vi "Open and Deploy RT Sequence blocking call.vi"(4 "Target (\"\": Auto-assign)":string, 5 "Timeout (ms)":dbl=10000.0, 6 "Gateway IP Address":string, 7 "Sequence File Path":path, 8 "ParamTypes":string[](array[string]), 9 "ParamValues":string[](array[string]), 10 "ParamNames":string[](array[string]), 11 "Sequence Context":refnum<k7>) -> (0 "error out":errorcluster, 2 "Report Text":string)   [LabVIEW 2015, in "RTSequenceVIs.lvlib"]
uses:
  RTSequenceVIs.lvlib
  <vilib>/NI Veristand/Execution/SequenceExecutionInterface/Sequence Execution State.ctl
  NationalInstruments.VeriStand.DataTypes
  <vilib>/NI Veristand/Execution/SequenceExecutionInterface/NI_VS Sequence Execution Interface.lvlib
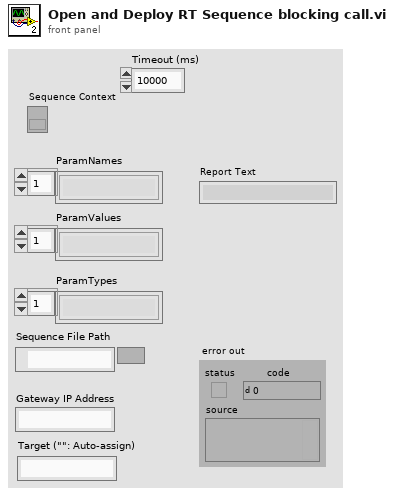
[diagram p1: front panel]
types:
  T1 = typedef "NI_VS Sequence Execution Interface.lvlib/Sequence Input Assignment Ref.ctl" = refnum<k24>
  T2 = typedef "NI_VS Sequence Execution Interface.lvlib/Sequence Call Ref.ctl" = refnum<k24>
  T3 = typedef "NI_VS Sequence Execution Interface.lvlib/Stimulus Profile Session Ref.ctl" = refnum<k24>
  T4 = typedef "TestStand - Status Monitor.ctl" = cluster{"Sequence Context":refnum<k7>, "Execution":refnum<k7>, "Termination Monitor":refnum<k7>}
  T5 = typedef "NI_VS Sequence Execution Interface.lvlib/Sequence Execution State.ctl" = enum16{"Idle", "Running", "SingleStepping", "Paused", "Stopped"}
  T6 = typedef "NI_VS Sequence Execution Interface.lvlib/Data Value Ref.ctl" = refnum<k24>
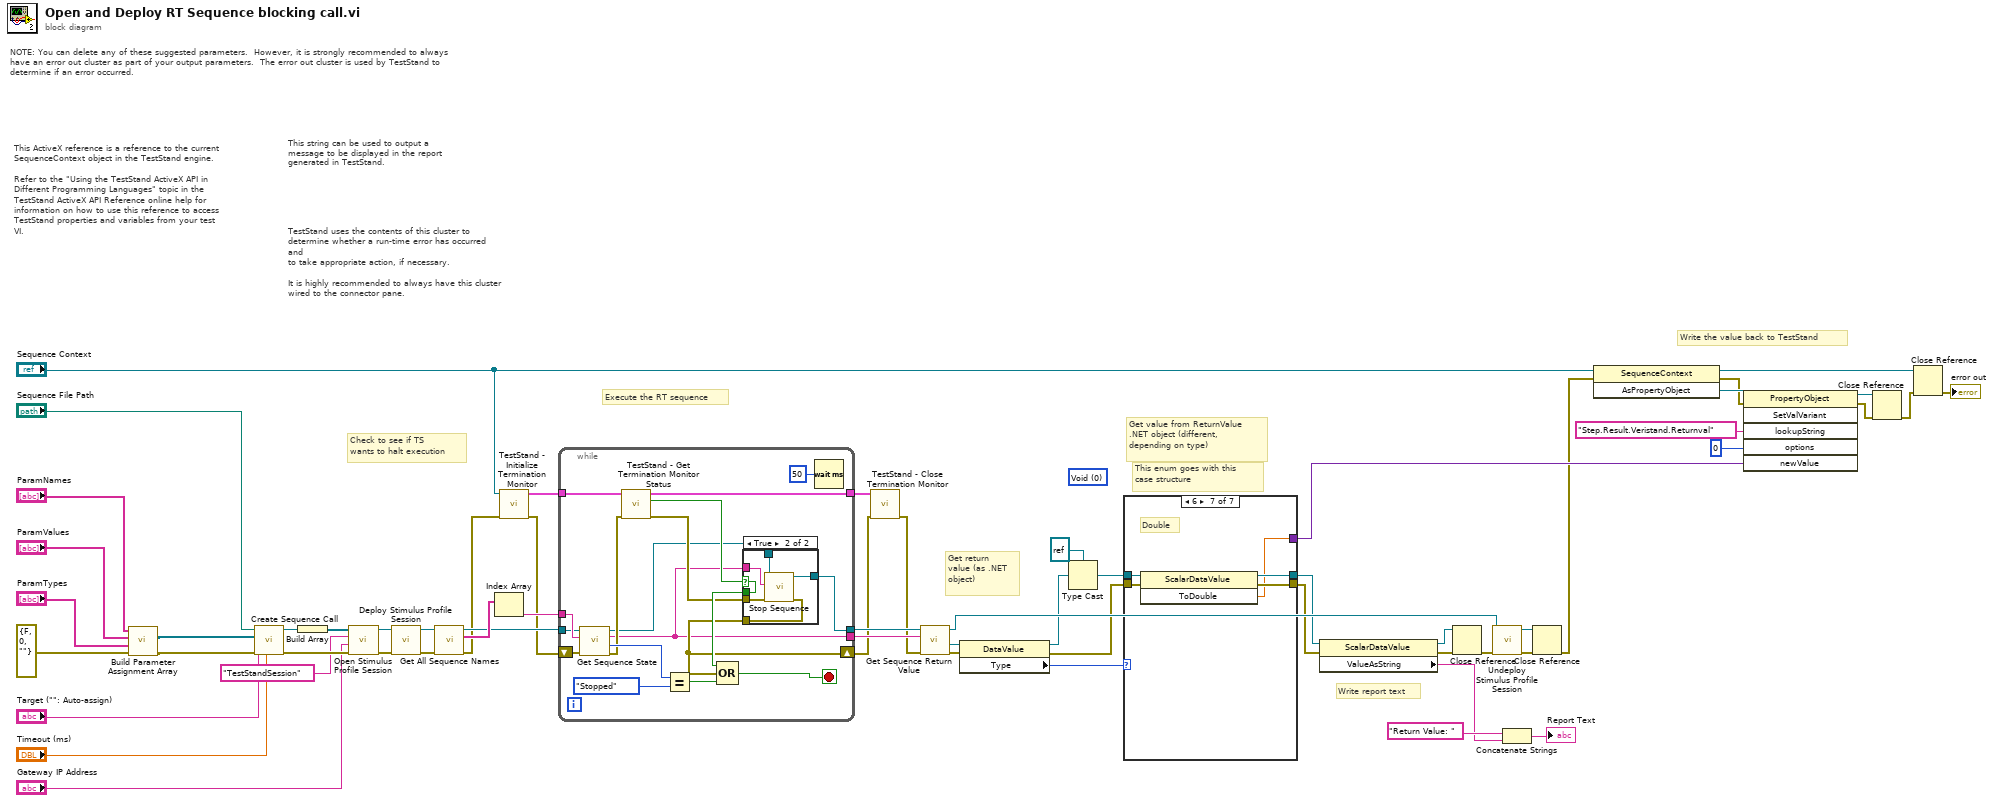
[diagram p0: block diagram]
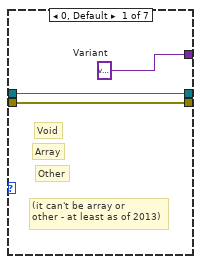
[diagram p2: hidden frame]
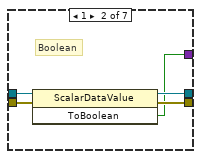
[diagram p3: hidden frame]
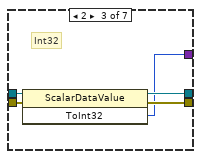
[diagram p4: hidden frame]
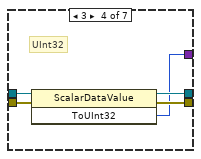
[diagram p5: hidden frame]
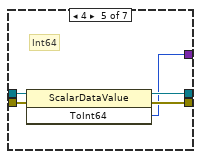
[diagram p6: hidden frame]
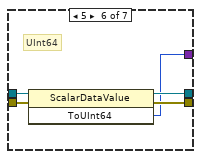
[diagram p7: hidden frame]
diagram:
  (unwired) 0 items=["Void", "Boolean", "Int32", "UInt32", "Int64", "UInt64", "Double", "Array"] ("Type")
  # "Check to see if TS\nwants to halt execution"
  # "Get value from ReturnValue\n.NET object (different, \ndepending on type)"
  # "Get return \nvalue (as .NET\nobject)"
  # "Write report text"
  # "Write the value back to TestStand"
  # "This enum goes with this \ncase structure"
  # "Execute the RT sequence"
  # "TestStand uses the contents of this cluster to\ndetermine whether a run-time error has occurred and\nto take appropriate action, if necessary.\n\nIt is highly recommended to always have this cluster\nwired to the connector pane."
  # "This string can be used to output a\nmessage to be displayed in the report\ngenerated in TestStand."
  # "NOTE: You can delete any of these suggested parameters.  However, it is strongly recommended to always have an error out cluster as part of your output parameters.  The error out cluster is used by TestStand to determine if an error occurred."
  # "This ActiveX reference is a reference to the current\nSequenceContext object in the TestStand engine.\n\nRefer to the \"Using the TestStand ActiveX API in\nDifferent Programming Languages\" topic in the \nTestStand ActiveX API Reference online help for\ninformation on how to use this reference to access\nTestStand properties and variables from your test VI."
  n1 = call "Build Parameter Assignment Array.vi"("error in (no error)"=errorcluster {"status"=FALSE, "code"=0, "source"=""}, "ParamTypes"="ParamTypes", "ParamValues"="ParamValues", "ParamNames"="ParamNames") -> ("error out"=w6:errorcluster, "Sequence Parameter Assignment refs"=w1:T1[])  [unwired: 6 in]
  n2 = call <vilib>:"Create Sequence Call.vi"("Timeout ms (10000)"="Timeout (ms)", "error in (no error)"=w6, "Target (\"\": Auto-assign)"="Target (\"\": Auto-assign)", "Parameter Assignments"=w1, "Sequence File Path"="Sequence File Path") -> ("error out"=w59:errorcluster, "Sequence Call Ref"=w53:T2)  [unwired: 5 in]
  n3 = Build Array(w53) -> (w57:T2[])
  n4 = call <vilib>:"Open Stimulus Profile Session.vi"("error in (no error)"=w59, "Gateway IP Address (\"\": localhost)"="Gateway IP Address", "Session Name"="TestStandSession", "Sequence Calls"=w57) -> ("error out"=w55:errorcluster, "Session Ref"=w56:T3)  [unwired: 6 in]
  n5 = call <vilib>:"Deploy Stimulus Profile Session.vi"("error in (no error)"=w55, "Session Ref in"=w56) -> ("error out"=w52:errorcluster, "Session Ref out"=w51:T3)  [unwired: 7 in, 1 out]
  n6 = call <vilib>:"Get All Sequence Names.vi"("error in (no error)"=w52, "Session Ref in"=w51) -> ("error out"=w15:errorcluster, "Sequence Names out"=w50:string[], "Session Ref out"=w48:T3)  [unwired: 7 in]
  n7 = Index Array(array=w50) -> (element=w49:string)  [unwired: 1 in]
  n8 = call <vilib>:"TestStand - Initialize Termination Monitor.vi"("error in (no error)"=w15, "Sequence Context In"="Sequence Context") -> ("error out"=w14:errorcluster, "Status Monitor Out"=w13:T4)  [unwired: 8 in]
  n9 = while {
    tunnel: w49 -> [w77]
    tunnel: w48 -> [w76]
    shift-right: [w63] -> w11
    shift-left: w14 -> [w75]
    tunnel: [w60] -> w44
    tunnel: [w62] -> w47
    tunnel: w13 -> [w69]
    tunnel: [w67] -> w12
    stop <- w71 stop-if-true
    n10 = call <vilib>:"Get Sequence State.vi"("error in (no error)"=w75, "Sequence Name"=w77, "Session Ref in"=w76) -> ("error out"=w68:errorcluster, "State"=w74:T5, "Sequence Name out"=w62:string, "Session Ref out"=w61:T3)  [unwired: 5 in]
    n11 = call <vilib>:"TestStand - Get Termination Monitor Status.vi"("error in (no error)"=w68, "Status Monitor In"=w69) -> ("error out"=w64:errorcluster, "Terminating or Aborting"=w66:bool, "Status Monitor Out"=w67:T4)  [unwired: 7 in]
    n12 = Equal?(x=w74, y=Sequence_Execution_State."Stopped" ("State")) -> (x = y?=w72:bool)
    n13 = case shown="True" w66 {
      selector: w66 -> [w80 w86]
      tunnel: [w80 w86] -> w65
      tunnel: w64 -> [w79 w85]
      tunnel: [w79 w84] -> w63
      tunnel: w62 -> [_ w83]
      tunnel: w61 -> [w78 w82]
      tunnel: [w78 w81] -> w60
      frame False {
      }
      frame True {
        n14 = call <vilib>:"Stop Sequence.vi"("error in (no error)"=w85, "Sequence Name"=w83, "Session Ref in"=w82) -> ("error out"=w84:errorcluster, "Session Ref out"=w81:T3)  [unwired: 6 in, 1 out]
      }
    }
    n15 = Compound Arithmetic op=OR(w65, w63, w72) -> (w71:bool)
    n16 = Wait (ms)(milliseconds to wait=u32 50 ("millisecond multiple")) -> ()  [unwired: 1 out]
  }
  n17 = call <vilib>:"TestStand - Close Termination Monitor.vi"("error in (no error)"=w11, "Status Monitor In"=w12) -> ("error out"=w10:errorcluster)  [unwired: 9 in]
  n18 = call <vilib>:"Get Sequence Return Value.vi"("error in (no error)"=w10, "Sequence Name"=w47, "Session Ref in"=w44) -> ("error out"=w38:errorcluster, "Data Value Ref"=w28:T6, "Session Ref out"=w43:T3)  [unwired: 5 in, 1 out]
  n19 = property class="DataValue"(reference=w28, error in=w38) -> (reference out=w36:T6, error out=w37:errorcluster, "Type"=w39:i32)
  n20 = Type Cast(type=refnum<k24> refnum ("Node"), x=w36) -> (*(type *) &x=w45:refnum<k24>)
  n21 = case shown="6" w39 {
    tunnel: w45 -> [w89 w94 w99 w104 w109 w114 w119]
    tunnel: [w88 w93 w97 w101 w106 w111 w116] -> w26
    tunnel: [w89 w92 w96 w102 w107 w112 w117] -> w27
    tunnel: w37 -> [w88 w91 w98 w103 w108 w113 w118]
    tunnel: [w87 w90 w95 w100 w105 w110 w115] -> w35
    frame 0, Default {
      w87 = variant  # Variant
      # "(it can't be array or \nother - at least as of 2013)"
      # "Other"
      # "Array"
      # "Void"
    }
    frame 1 {
      # "Boolean"
      n22 = invoke class="ScalarDataValue" method="ToBoolean"(reference=w94, error in=w91) -> (reference out=w92:refnum<k24>, error out=w93:errorcluster, "ToBoolean"=w90:bool)  [unwired: 1 in]
    }
    frame 2 {
      # "Int32"
      n23 = invoke class="ScalarDataValue" method="ToInt32"(reference=w99, error in=w98) -> (reference out=w96:refnum<k24>, error out=w97:errorcluster, "ToInt32"=w95:i32)  [unwired: 1 in]
    }
    frame 3 {
      # "UInt32"
      n24 = invoke class="ScalarDataValue" method="ToUInt32"(reference=w104, error in=w103) -> (reference out=w102:refnum<k24>, error out=w101:errorcluster, "ToUInt32"=w100:u32)  [unwired: 1 in]
    }
    frame 4 {
      # "Int64"
      n25 = invoke class="ScalarDataValue" method="ToInt64"(reference=w109, error in=w108) -> (reference out=w107:refnum<k24>, error out=w106:errorcluster, "ToInt64"=w105:i64)  [unwired: 1 in]
    }
    frame 5 {
      # "UInt64"
      n26 = invoke class="ScalarDataValue" method="ToUInt64"(reference=w114, error in=w113) -> (reference out=w112:refnum<k24>, error out=w111:errorcluster, "ToUInt64"=w110:u64)  [unwired: 1 in]
    }
    frame 6 {
      # "Double"
      n27 = invoke class="ScalarDataValue" method="ToDouble"(reference=w119, error in=w118) -> (reference out=w117:refnum<k24>, error out=w116:errorcluster, "ToDouble"=w115:dbl)  [unwired: 1 in]
    }
  }
  n28 = property class="ScalarDataValue"(reference=w27, error in=w26) -> (reference out=w25:refnum<k24>, error out=w24:errorcluster, "ValueAsString"=w17:string)
  n29 = Close Reference(reference=w25, error in (no error)=w24) -> (error out=w42:errorcluster)
  n30 = call <vilib>:"Undeploy Stimulus Profile Session.vi"("error in (no error)"=w42, "Session Ref in"=w43) -> ("error out"=w23:errorcluster, "Session Ref out"=w22:T3)  [unwired: 8 in]
  n31 = Concatenate Strings("Return Value: ", w17) -> (→"Report Text":string)
  n32 = Close Reference(reference=w22, error in (no error)=w23) -> (error out=w21:errorcluster)
  n33 = invoke class="SequenceContext" method="AsPropertyObject"(reference="Sequence Context", error in=w21) -> (reference out=w32:refnum<k7>, error out=w30:errorcluster, "AsPropertyObject"=w41:refnum<k7>)  [unwired: 1 in]
  n34 = invoke class="PropertyObject" method="SetValVariant"(reference=w41, error in=w30, "lookupString"="Step.Result.Veristand.Returnval", "options"=0, "newValue"=w35) -> (reference out=w34:refnum<k7>, error out=w33:errorcluster)  [unwired: 1 in, 4 out]
  n35 = Close Reference(reference=w34, error in (no error)=w33) -> (error out=w31:errorcluster)
  n36 = Close Reference(reference=w32, error in (no error)=w31) -> (error out=→"error out":errorcluster)
